vi "commandEnterMaintenance.vi"(8 "error in (no error)":errorcluster, 10 "CommandEnterMaintenance in":T1, 11 "Communicator in":refnum<class "Communicator.lvclass">) -> (0 "error out":errorcluster, 2 "CommandEnterMaintenance out":T1, 3 "Communicator out":refnum<class "Communicator.lvclass">)   [LabVIEW 2016, in "M1M3SupportCommunicator.lvlib" / "Communicator.lvclass"]
uses:
  Communicator.lvclass
  DataTypes/Topics/CommandEnterMaintenance.ctl
  DataTypes/Topics/Parts/CommandId.ctl
  DataTypes/Topics/M1M3SupportTopics.lvlib
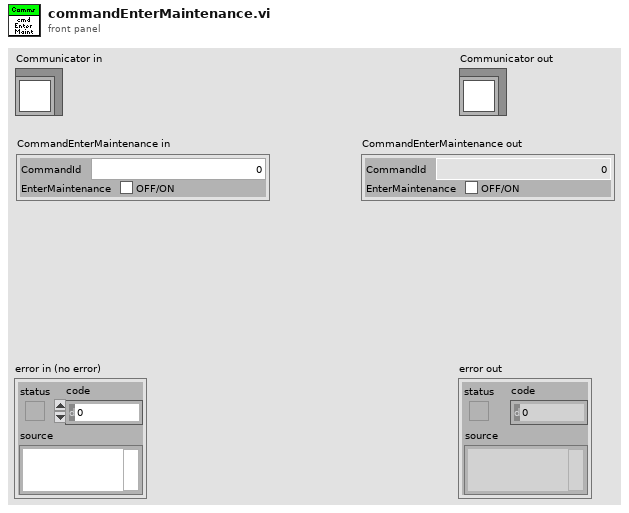
[diagram p1: front panel]
types:
  T1 = typedef "M1M3SupportTopics.lvlib/CommandEnterMaintenance.ctl" = cluster{"CommandId":T2, "EnterMaintenance":bool}
  T2 = typedef "M1M3SupportTopics.lvlib/CommandId.ctl" = i32
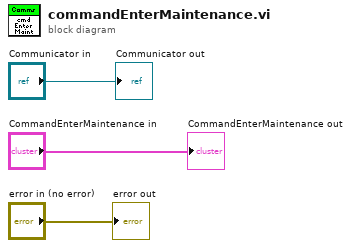
[diagram p0: block diagram]
diagram:
  "error out" <- "error in (no error)"
  "Communicator out" <- "Communicator in"
  "CommandEnterMaintenance out" <- "CommandEnterMaintenance in"
